vi "SignFromKeybordEvent.vi"() -> ()   [LabVIEW 2020]
doc: "Read pressed keybord button. Comments in english and polish language."
panel:
  out "Sign":string
  in  "stop":bool
  out "ASCII Code Dec":i16
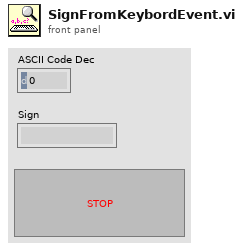
[diagram p1: front panel]
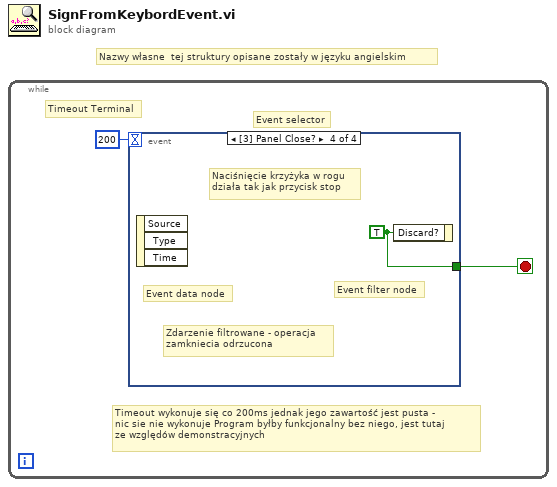
[diagram p0: block diagram]
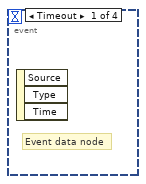
[diagram p2: hidden frame]
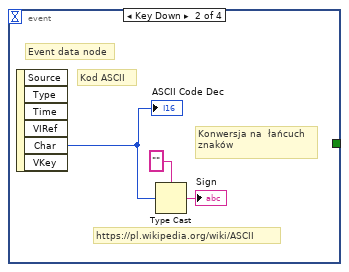
[diagram p3: hidden frame]
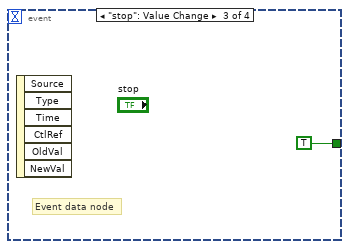
[diagram p4: hidden frame]
diagram:
  # "Nazwy własne  tej struktury opisane zostały w języku angielskim"
  n1 = while {
    stop <- w2 stop-if-true
    # "Timeout wykonuje się co 200ms jednak jego zawartość jest pusta -\nnic sie nie wykonuje Program byłby funkcjonalny bez niego, jest tutaj\nze względów demonstracyjnych"
    # "Event selector"
    # "Timeout Terminal"
    n2 = event shown="[3] Panel Close?" {
      selector: _ -> [_ _ _ _]
      dyn-events: _ -> [_ _ _ _]
      timeout: 200 -> [_ _ _ _]
      tunnel: [_ _ TRUE w7] -> w2
      event Timeout {
        # "Event data node"
        n3 = event-data() -> ()  [unwired: 1 in, 3 out]
      }
      event Key Down {
        # "https://pl.wikipedia.org/wiki/ASCII"
        # "Konwersja na  łańcuch\nznaków"
        # "Kod ASCII"
        # "Event data node"
        n4 = event-data() -> ("Char"=w5:i16)  [unwired: 1 in, 5 out]
        "ASCII Code Dec" <- w5
        n5 = Type Cast(type="", x=w5) -> (*(type *) &x=→"Sign":string)
      }
      event "stop": Value Change {
        # "Event data node"
        n6 = event-data() -> ()  [unwired: 1 in, 6 out]
      }
      event Panel Close? {
        w7 = TRUE ("Discard?")
        # "Zdarzenie filtrowane - operacja \nzamkniecia odrzucona"
        # "Naciśnięcie krzyżyka w rogu\ndziała tak jak przycisk stop"
        # "Event filter node"
        # "Event data node"
        n7 = event-data() -> ()  [unwired: 1 in, 3 out]
        n8 = event-data("Discard?"=w7) -> ()  [unwired: 1 in, 1 out]
      }
    }
  }
